vi "SimpleScanning_August12_2016.vi"() -> ()   [LabVIEW 2010]
uses:
  <vilib>/DAQmx/configure/timing.llb/DAQmx Timing (Sample Clock).vi
  <vilib>/Analysis/NI_AALBase.lvlib
  <vilib>/DAQmx/create/channels.llb/DAQmx Create Channel (AO-Voltage-Basic).vi
  <vilib>/DAQmx/configure/trigger.llb/DAQmx Start Trigger (Digital Edge).vi
  <vilib>/DAQmx/create/channels.llb/DAQmx Create Channel (AI-Voltage-Basic).vi
  <vilib>/DAQmx/read.llb/DAQmx Read (Analog 1D DBL 1Chan NSamp).vi
  <vilib>/DAQmx/write.llb/DAQmx Write (Analog 2D DBL NChan NSamp).vi
panel:
  in  "offset (V)":dbl=1000.0
  in  "display scaled image?":bool
  in  "Pixels (X,Y)":i32[](array[numeric])=[200, 200]
  in  "Scan amplitude (X,Y) (V)":dbl[](array[numeric])=[2.0, 2.0]
  out "min,max raw pixel voltage":dbl[](array[numeric])
  in  "scale factor":i32=1000
  in  "rescale pixel values":bool=TRUE
  out "Histogram Graph":T1(graph)
  out "Image Gr":dbl[][](graph)
  in  "Invert":bool=TRUE
  out "file path":path
  out "file #":i32
  in  "file tag":string="t"
  out "stop 2":bool
  in  "SAVE":bool
  in  "AI input\nconfiguration":i32(ring)=-1 items=["default"=-1, "RSE"=10083, "NRSE"=10078, "Differential"=10106, "Pseudodifferential"=12529]
  in  "refnum tif":refnum<file>
  in  "AI range (+/-) (V)":dbl=2.0 format="%#_13g"
  in  "AI rate (Hz): Max":dbl=4000000.0 format="%#_13g"
  in  "AO rate (Hz): Max":dbl=4000000.0 format="%#_13g"
  out "Array":dbl[][](array[numeric])
  out "Saved":i32
  in  "save local":bool
  in  "#frames":i32=10
  in  "Data Folder":path=path "C:/Users/TENSS/Desktop"
  out "Ypixels":i32=200
  in  "bidirectional":bool
  in  "samples to bin":i32=5
  out "current AI Rate (Hz)":dbl=2500000.0 format="%0.2f"
  in  "y flyback":bool=TRUE
  in  "stop":bool
  out "xy scan waveform":dbl[][](array[numeric])
  out "dwell time [us]":dbl=2.0
  in  "pixel shift":i32
  out "chunk to read":i32=1400
  out "input buffer size":i32=5000000
  in  "reset":bool
  out "#samples/frame":i32=56280
  out "Frame rate (hz)":dbl=8.884150675195452
  out "nlines":i32=200
  in  "flyback pixels (X)":i32=80
  out "Xpixels":i32=200
  in  "current AO Rate (Hz)":dbl=50000.0 format="%0.2f"
  # "Scan and Image assembly"
  # "DAQ related settings"
  # "Adjust scale factor, invert  to ensure the histogram\nspans large range 0-10000 or more\n--- efficiently use of the 16 bit dynamic range"
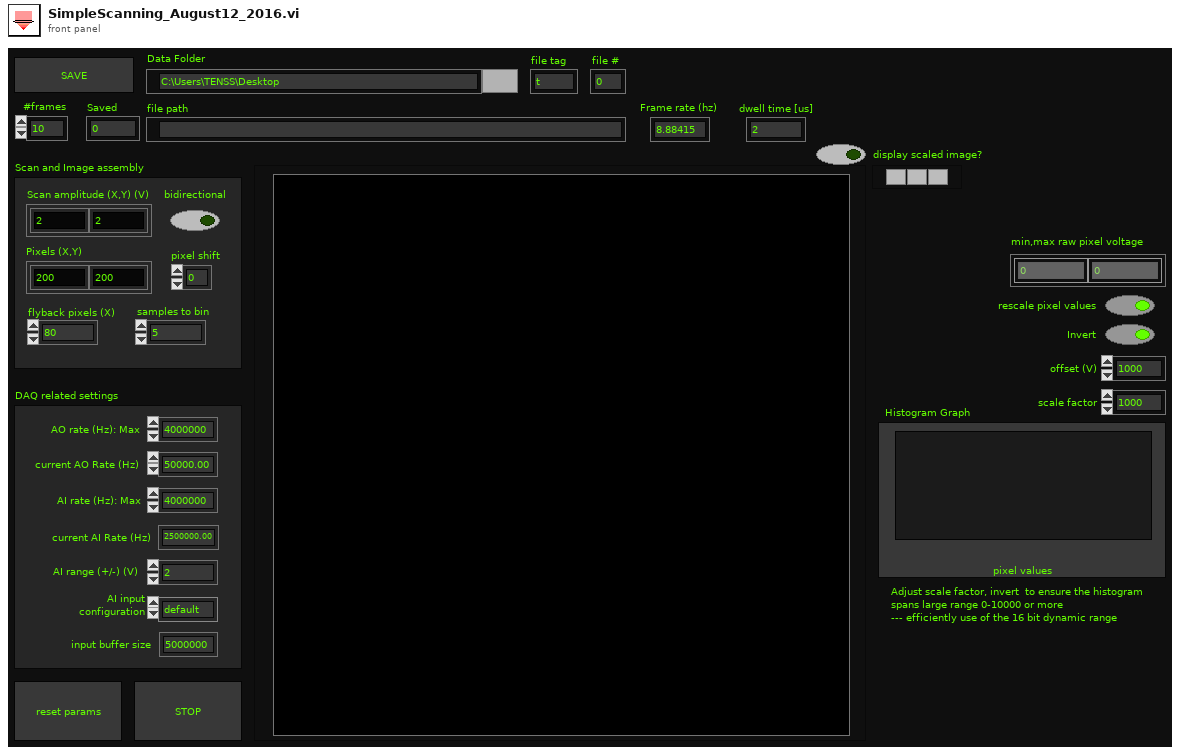
[diagram p1: front panel]
types:
  T1 = cluster{"X Values":dbl[], "Histogram: h(x)":i32[]}
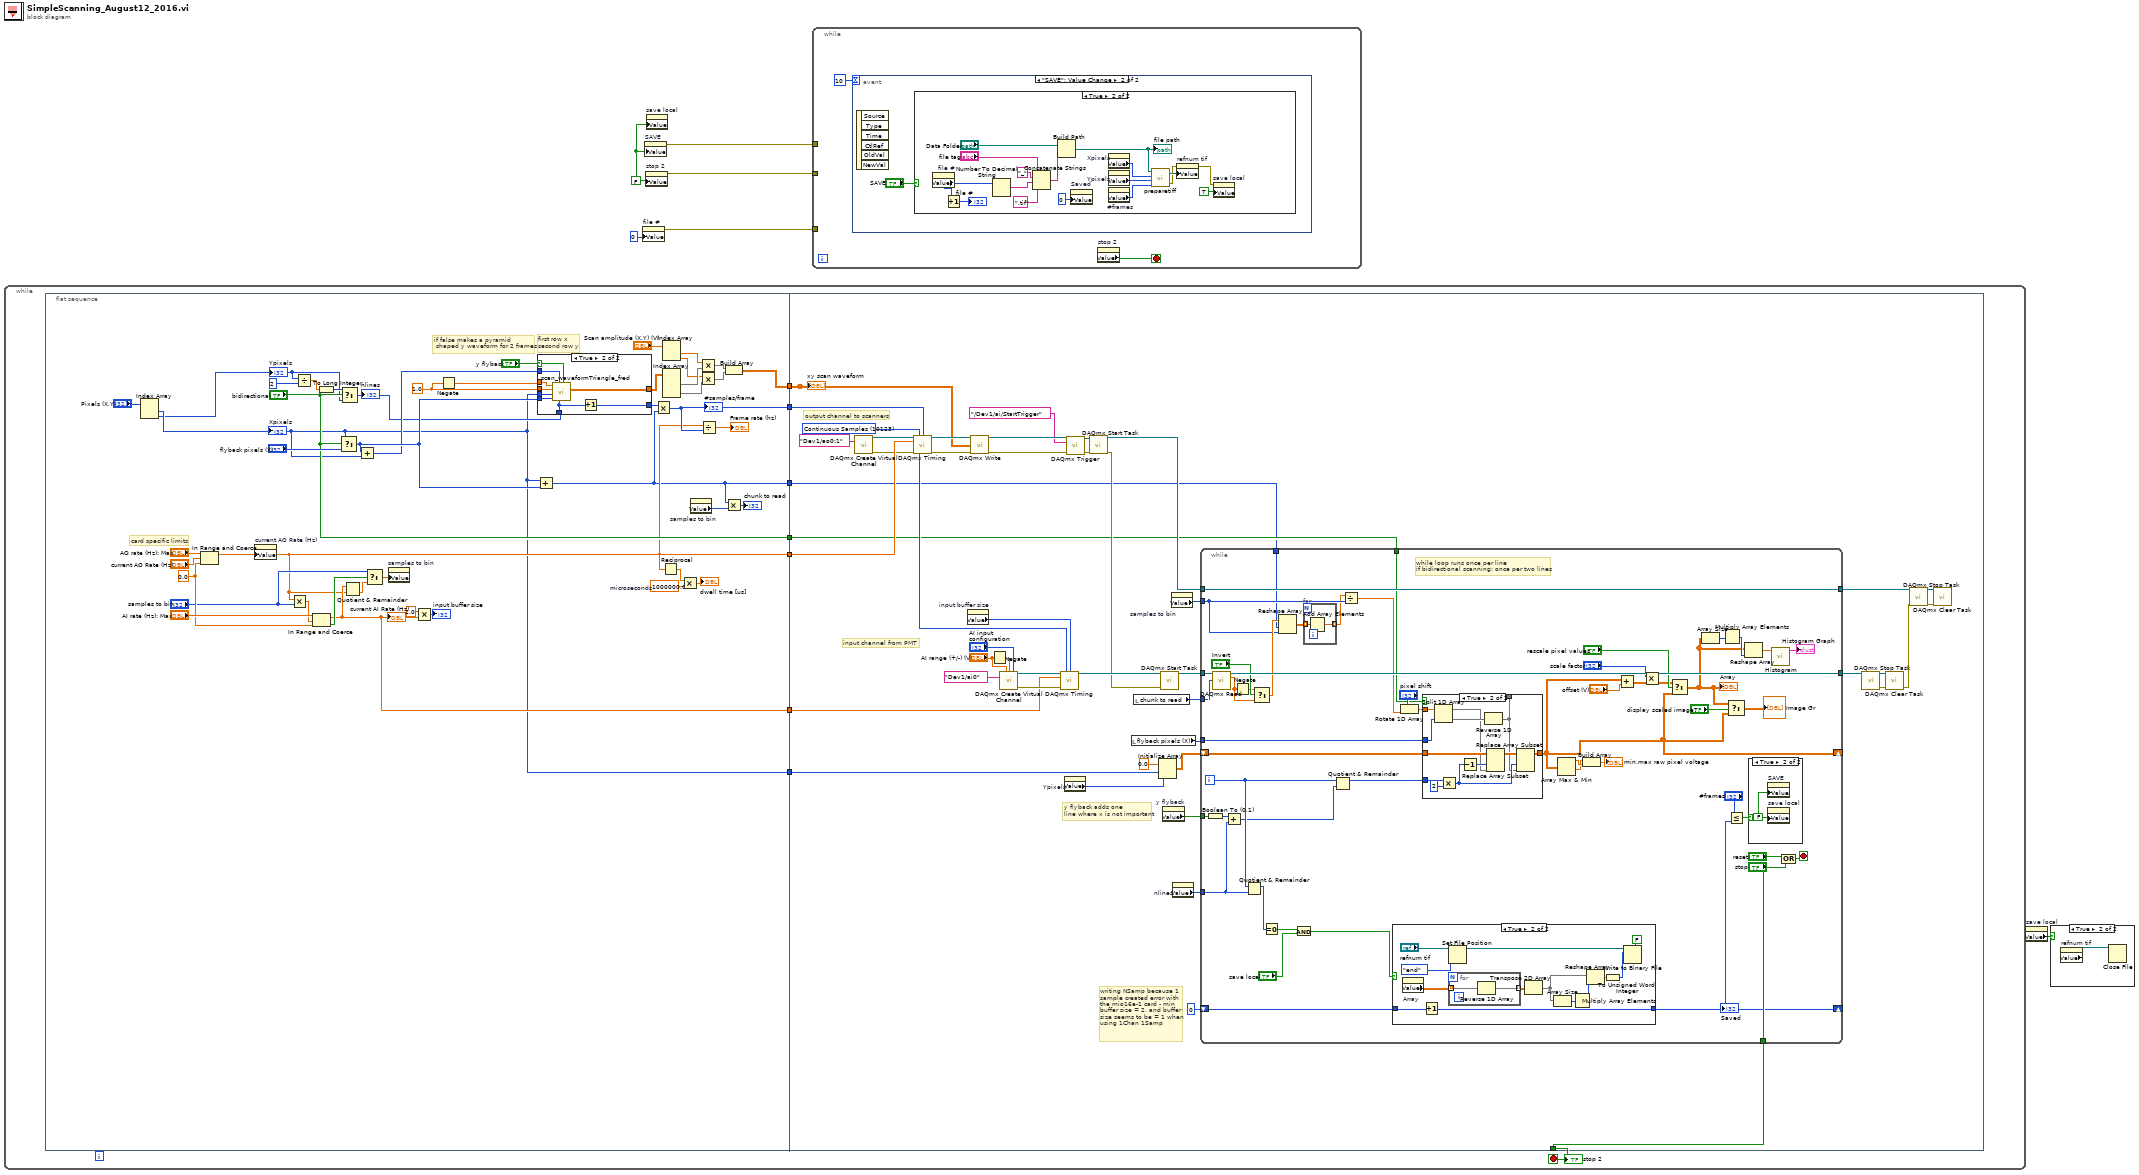
[diagram p0: block diagram]
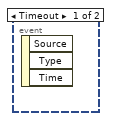
[diagram p2: hidden frame]
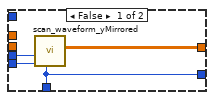
[diagram p5: hidden frame]
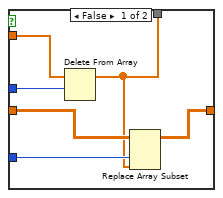
[diagram p8: hidden frame]
diagram:
  w4 = FALSE ("stop 2")
  n1 = while {
    stop <- w14 stop-if-true
    n2 = flat-sequence {
      tunnel: [w25] -> w13
      tunnel: [w43] -> w12
      tunnel: [w15] -> w11
      tunnel: [w29] -> w10
      tunnel: [w31] -> w9
      tunnel: ["bidirectional"] -> w8
      tunnel: [w28] -> w7
      tunnel: [w105] -> w14
      tunnel: w13 -> [w89]
      tunnel: w12 -> [w88]
      tunnel: w11 -> [w73]
      tunnel: w10 -> [w87]
      tunnel: w9 -> [w85]
      tunnel: w8 -> [w84]
      tunnel: w7 -> [w74]
      frame #0 {
        w27 = 1.0 ("scan voltage")
        w38 = 0.0 ("lower limit")
        w45 = 1000000.0  # microseconds
        # "card specific limits"
        # "first row x\nsecond row y"
        # "if false makes a pyramid\n shaped y waveform for 2 frames"
        n3 = Index Array(array="Pixels (X,Y)") -> (element #1=w25:i32, element #2=w24:i32)  [unwired: 2 in]
        "Xpixels" <- w25
        "Ypixels" <- w24
        n4 = In Range and Coerce(upper limit="AO rate (Hz): Max", x="current AO Rate (Hz)", lower limit=w38) -> (coerced(x)=w29:dbl)  [unwired: 1 out]
        n5 = property on="current AO Rate (Hz)" class="DigNum (strict)"("Value"=w29) -> ()  [unwired: 2 in, 2 out]
        n6 = Multiply(x=w29, y="samples to bin") -> (x*y=w37:dbl)
        n7 = Divide(x=w24, y=2) -> (x/y=w52:dbl)
        n8 = In Range and Coerce(upper limit="AI rate (Hz): Max", x=w37, lower limit=w38) -> (coerced(x)=w31:dbl, In Range?=w36:bool)
        "current AI Rate (Hz)" <- w31
        n9 = To Long Integer(number=w52) -> (32bit integer=w47:i32)
        n10 = Select(t=w25, s="bidirectional", f="flyback pixels (X)") -> (s? t:f=w50:i32)
        n11 = Select(t=w47, s="bidirectional", f=w24) -> (s? t:f=w48:i32)
        "nlines" <- w48
        n12 = Quotient & Remainder(x=w31, y=w29) -> (floor(x/y)=w34:dbl)  [unwired: 1 out]
        n13 = Add(x=w50, y=w25) -> (x+y=w49:i32)
        n14 = Select(t="samples to bin", s=w36, f=w34) -> (s? t:f=w33:dbl)
        n15 = property on="samples to bin" class="DigNum (strict)"("Value"=w33) -> ()  [unwired: 2 in, 2 out]
        n16 = Multiply(x=2.0 ("y"), y=w31) -> (x*y=→"input buffer size":dbl)
        n17 = Negate(x=w27) -> (-x=w55:dbl)
        n18 = case shown="True" "y flyback" {
          selector: "y flyback" -> [_ w66]
          tunnel: w48 -> [w60 w65]
          tunnel: [w63 w70] -> w23
          tunnel: w50 -> [w62 w72]
          tunnel: w25 -> [w61 w71]
          tunnel: w55 -> [_ w69]
          tunnel: w27 -> [_ w68]
          tunnel: w49 -> [_ w67]
          tunnel: [w60 w64] -> w46
          frame False {
            n19 = call "scan_waveform_yMirrored.vi"("nlines"=w60, "flyback"=w62, "xpixels"=w61) -> ("xy scan waveform"=w63:dbl[][])  [unwired: 4 in, 4 out]
          }
          frame True {
            n20 = call "scan_waveformTriangle_fred.vi"(5:"y flyback"=w66, "nlines"=w65, 7:"y flyback"=w67, "flyback"=w72, "xpixels"=w71, "maxV"=w68, "minV"=w69) -> ("xy scan waveform"=w70:dbl[][])  [unwired: 4 out]
            n21 = Increment(x=w65) -> (x+1=w64:i32)
          }
        }
        n22 = Add(x=w25, y=w50) -> (x+y=w28:i32)
        n23 = Multiply(x=w46, y=w28) -> (x*y=w43:i32)
        "#samples/frame" <- w43
        n24 = Reciprocal(x=w29) -> (1/x=w32:dbl)
        n25 = Index Array(array="Scan amplitude (X,Y) (V)") -> (element #1=w21:dbl, element #2=w18:dbl)  [unwired: 2 in]
        n26 = Index Array(array=w23) -> (element #1=w19:dbl[], element #2=w20:dbl[])  [unwired: 4 in]
        n27 = Multiply(x=w32, y=w45) -> (x*y=→"dwell time [us]":dbl)
        n28 = property on="samples to bin" class="DigNum (strict)"() -> ("Value"=w44:i32)  [unwired: 2 in, 2 out]
        n29 = Multiply(x=w21, y=w19) -> (x*y=w17:dbl[])
        n30 = Multiply(x=w18, y=w20) -> (x*y=w16:dbl[])
        n31 = Divide(x=w29, y=w43) -> (x/y=→"Frame rate (hz)":dbl)
        n32 = Build Array(w17, w16) -> (w15:dbl[][])
        n33 = Multiply(x=w28, y=w44) -> (x*y=→"chunk to read":i32)
      }
      frame #1 {
        w86 = 10123 items=["Finite Samples"=10178, "Continuous Samples"=10123, "Hardware Timed Single Point"=12522] ("sample mode")
        # "writing NSamp because 1 sample created error with\nthe mio16e-1 card - min\nbuffer size = 2, and buffer size seems to be = 1 when using 1Chan 1Samp"
        # "y flyback adds one\nline where x is not important"
        # "input channel from PMT"
        # "output channel to scanners"
        n34 = call-poly <vilib>:"DAQmx Create Virtual Channel.vi"("physical channels"=tag "Dev1/ao0:1") -> ("task out"=w79:refnum<k21>, "error out"=w78:errorcluster)  [unwired: 13 in]
        n35 = call-poly <vilib>:"DAQmx Timing.vi"("task/channels in"=w79, "sample mode"=w86, "samples per channel"=w88, "rate"=w87, "error in"=w78) -> ("task out"=w118:refnum<k21>, "error out"=w103:errorcluster)  [unwired: 2 in, 7 out]
        n36 = property on="input buffer size" class="DigNum (strict)"() -> ("Value"=w96:i32)  [unwired: 2 in, 2 out]
        n37 = call-poly <vilib>:"DAQmx Write.vi"("task/channels in"=w118, "data"=w73, "error in"=w103) -> ("task out"=w102:refnum<k21>, "error out"=w100:errorcluster)  [unwired: 1 in, 10 out]
        n38 = Negate(x="AI range (+/-) (V)") -> (-x=w90:dbl)
        n39 = call-poly <vilib>:"DAQmx Create Virtual Channel.vi"("maximum value"="AI range (+/-) (V)", "minimum value"=w90, "input terminal configuration"="AI input\nconfiguration", "physical channels"=tag "Dev1/ai0") -> ("task out"=w114:refnum<k21>, "error out"=w113:errorcluster)  [unwired: 5 in, 5 out]
        n40 = call-poly <vilib>:"DAQmx Timing.vi"("task/channels in"=w114, "sample mode"=w86, "samples per channel"=w96, "rate"=w85, "error in"=w113) -> ("task out"=w112:refnum<k21>)  [unwired: 2 in, 8 out]
        n41 = property on="Ypixels" class="DigNum (strict)"() -> ("Value"=w94:i32)  [unwired: 2 in, 2 out]
        n42 = call-poly <vilib>:"DAQmx Trigger.vi"("task/channels in"=w102, "source"=tag "/Dev1/ai/StartTrigger", "error in"=w100) -> ("task out"=w101:refnum<k21>, "error out"=w99:errorcluster)  [unwired: 1 in, 10 out]
        n43 = call <vilib>:"DAQmx Start Task.vi"("task/channels in"=w101, "error in"=w99) -> ("task out"=w117:refnum<k21>, "error out"=w98:errorcluster)  [unwired: 12 out]
        n44 = local read "flyback pixels (X)"() -> (w95:i32)
        n45 = local read "chunk to read"() -> (w106:i32)
        n46 = Initialize Array(0.0 ("element"), w89, w94) -> (w107:dbl[][])
        n47 = call <vilib>:"DAQmx Start Task.vi"("task/channels in"=w112, "error in"=w98) -> ("task out"=w111:refnum<k21>)  [unwired: 13 out]
        n48 = property on="y flyback" class="Bool (strict)"() -> ("Value"=w104:bool)  [unwired: 2 in, 2 out]
        n49 = property on="samples to bin" class="DigNum (strict)"() -> ("Value"=w97:i32)  [unwired: 2 in, 2 out]
        n50 = property on="nlines" class="DigNum (strict)"() -> ("Value"=w93:i32)  [unwired: 2 in, 2 out]
        n51 = while {
          tunnel: w117 -> [w169]
          tunnel: [w169] -> w116
          tunnel: w111 -> [w168]
          tunnel: [w167] -> w109
          tunnel: w106 -> [w166]
          tunnel: w95 -> [w165]
          shift-right: [w124] -> _
          shift-left: w107 -> [w157]
          tunnel: w93 -> [w148]
          tunnel: ["stop"] -> w105
          tunnel: w104 -> [w160]
          tunnel: w97 -> [w135]
          tunnel: w84 -> [w158]
          shift-right: [w155] -> _
          shift-left: 0 ("Border Size") -> [w156]
          tunnel: w74 -> [w134]
          i -> [w153]
          stop <- w163 stop-if-true
          # "while loop runs once per line\nif bidirectional scanning: once per two lines"
          n52 = Boolean To (0,1)(Boolean=w160) -> (0, 1=w150:i16)
          n53 = call-poly <vilib>:"DAQmx Read.vi"("task/channels in"=w168, "number of samples per channel"=w166) -> ("task out"=w167:refnum<k21>, "data"=w137:dbl[])  [unwired: 1 in, 11 out]
          n54 = Add(x=w150, y=w148) -> (x+y=w149:i32)
          n55 = Negate(x=w137) -> (-x=w144:dbl[])
          n56 = Quotient & Remainder(x=w153, y=w148) -> (x-y*floor(x/y)=w152:i32)  [unwired: 1 out]
          n57 = Select(t=w144, s="Invert", f=w137) -> (s? t:f=w136:dbl[])
          n58 = Equal To 0?(x=w152) -> (x = 0?=w129:bool)
          n59 = Reshape Array(w136, w134, w135) -> (w133:dbl[][])
          n60 = And(x=w129, y="save local") -> (x .and. y?=w126:bool)
          n61 = for {
            tunnel: w133 -> [w187] mode=indexing
            tunnel: [w186] -> w132 mode=indexing
            n62 = Add Array Elements(numeric array=w187) -> (sum=w186:dbl)
          }
          n63 = Quotient & Remainder(x=w153, y=w149) -> (x-y*floor(x/y)=w154:i32)  [unwired: 1 out]
          n64 = Divide(x=w132, y=w135) -> (x/y=w145:dbl[])
          n65 = case shown="True" w126 {
            tunnel: w156 -> [w170 w180]
            tunnel: [w170 w179] -> w155
            frame False {
            }
            frame True {
              n66 = property on="Array" class="Arr (strict)"() -> ("Value"=w171:dbl[][])  [unwired: 2 in, 2 out]
              n67 = Increment(x=w180) -> (x+1=w179:i32)
              n68 = Set File Position(refnum="refnum tif", from (0:start)=enum16{"start", "end", "current"}."end") -> (refnum out=w183:refnum<file>)  [unwired: 1 in, 2 out]
              n69 = for {
                tunnel: w171 -> [w185] mode=indexing
                tunnel: [w184] -> w173 mode=indexing
                n70 = Reverse 1D Array(array=w185) -> (reversed array=w184:dbl[])
              }
              n71 = Transpose 2D Array(2D array=w173) -> (transposed array=w172:dbl[][])
              n72 = Array Size(array=w172) -> (size(s)=w178:i32[])
              n73 = Multiply Array Elements(1:w178) -> (0:w177:i32)
              n74 = Reshape Array(w172, w177) -> (w176:dbl[])
              n75 = To Unsigned Word Integer(number=w176) -> (unsigned 16bit integer=w175:u16[])
              n76 = Write to Binary File(file (use dialog)=w183, data=w175, 5:FALSE ("prepend array or string size? (T)")) -> ()  [unwired: 2 in, 4 out]
            }
          }
          "Saved" <- w155
          n77 = Rotate 1D Array(1:w145, 2:"pixel shift") -> (0:w164:dbl[])
          n78 = case shown="True" w158 {
            tunnel: w165 -> [w194 w204]
            tunnel: w164 -> [w193 w206]
            tunnel: w157 -> [w192 w201]
            tunnel: [w191 w197] -> w124
            tunnel: w154 -> [w190 w202]
            tunnel: [w189 w195] -> _
            frame False {
              n79 = Delete From Array(array=w193, length=w194) -> (array with subset deleted=w189:dbl[])  [unwired: 1 in, 1 out]
              n80 = Replace Array Subset(array=w192, new element=w189, index (col)=w190) -> (w191:dbl[][])  [unwired: 1 in]
            }
            frame True {
              n81 = Split 1D Array(array=w206, index=w204) -> (first subarray=w196:dbl[], second subarray=w205:dbl[])
              n82 = Multiply(x=w202, y=2) -> (x*y=w198:i32)
              n83 = Decrement(x=w198) -> (x-1=w200:i32)
              n84 = Reverse 1D Array(array=w205) -> (reversed array=w195:dbl[])
              n85 = Replace Array Subset(array=w201, new element=w196, index (col)=w200) -> (w199:dbl[][])  [unwired: 1 in]
              n86 = Replace Array Subset(array=w199, new element=w195, index (col)=w198) -> (w197:dbl[][])  [unwired: 1 in]
            }
          }
          n87 = Array Max & Min(array=w124) -> (max value=w120:dbl, min value=w119:dbl)  [unwired: 2 out]
          n88 = Build Array(w119, w120) -> (→"min,max raw pixel voltage":dbl[])
          n89 = Add(x=w124, y="offset (V)") -> (x+y=w138:dbl[][])
          n90 = Multiply(x="scale factor", y=w138) -> (x*y=w125:dbl[][])
          n91 = Select(t=w125, s="rescale pixel values", f=w124) -> (s? t:f=w123:dbl[][])
          "Array" <- w123
          n92 = Array Size(array=w123) -> (size(s)=w141:i32[])
          n93 = Multiply Array Elements(1:w141) -> (0:w140:i32)
          n94 = Select(t=w123, s="display scaled image?", f=w124) -> (s? t:f=→"Image Gr":dbl[][])
          n95 = Less Or Equal?(x="#frames", y=w155) -> (x <= y?=w147:bool)
          n96 = Reshape Array(w123, w140) -> (w139:dbl[])
          n97 = case shown="True" w147 {
            frame False {
            }
            frame True {
              w188 = FALSE
              n98 = property on="SAVE" class="Bool (strict)"("Value"=w188) -> ()  [unwired: 2 in, 2 out]
              n99 = property on="save local" class="Bool (strict)"("Value"=w188) -> ()  [unwired: 2 in, 2 out]
            }
          }
          n100 = call <vilib>:"Histogram.vi"("X"=w139) -> ("Histogram Graph"=→"Histogram Graph":T1)  [unwired: 7 in, 3 out]
          n101 = Compound Arithmetic op=OR("reset", "stop") -> (w163:bool)
        }
        n102 = call <vilib>:"DAQmx Stop Task.vi"("task/channels in"=w109) -> ("task out"=w110:refnum<k21>, "error out"=w83:errorcluster)  [unwired: 1 in, 12 out]
        n103 = call <vilib>:"DAQmx Clear Task.vi"("task in"=w110, "error in"=w83) -> ("error out"=w82:errorcluster)  [unwired: 13 out]
        n104 = call <vilib>:"DAQmx Stop Task.vi"("task/channels in"=w116, "error in"=w82) -> ("task out"=w115:refnum<k21>, "error out"=w81:errorcluster)  [unwired: 12 out]
        n105 = call <vilib>:"DAQmx Clear Task.vi"("task in"=w115, "error in"=w81) -> ()  [unwired: 14 out]
        "xy scan waveform" <- w73
      }
    }
    "stop 2" <- w14
  }
  n106 = property on="file #" class="DigNum (strict)"("Value"=0 ("file number")) -> (error out=w2:errorcluster)  [unwired: 2 in, 1 out]
  n107 = property on="SAVE" class="Bool (strict)"("Value"=w4) -> (error out=w3:errorcluster)  [unwired: 2 in, 1 out]
  n108 = property on="stop 2" class="Bool (strict)"("Value"=w4) -> (error out=w1:errorcluster)  [unwired: 2 in, 1 out]
  n109 = property on="save local" class="Bool (strict)"("Value"=w4) -> ()  [unwired: 2 in, 2 out]
  n110 = while {
    tunnel: w3 -> [_]
    tunnel: w2 -> [_]
    tunnel: w1 -> [_]
    stop <- w207 stop-if-true
    n111 = event shown="[1] \"SAVE\": Value Change" {
      selector: _ -> [_ _]
      dyn-events: _ -> [_ _]
      timeout: 10 -> [_ _]
      event Timeout {
        n112 = event-data() -> ()  [unwired: 1 in, 3 out]
      }
      event "SAVE": Value Change {
        n113 = event-data() -> ()  [unwired: 1 in, 6 out]
        n114 = case shown="True" "SAVE" {
          frame False {
          }
          frame True {
            n115 = property on="file #" class="DigNum (strict)"() -> ("Value"=w211:i32)  [unwired: 2 in, 2 out]
            n116 = Increment(x=w211) -> (x+1=→"file #":i32)
            n117 = Number To Decimal String(number=w211) -> (decimal integer string=w219:string)  [unwired: 1 in]
            n118 = Concatenate Strings("file tag", "_" ("string"), w219, ".tif" ("string")) -> (w215:string)
            n119 = Build Path(base path="Data Folder", name or relative path=w215) -> (appended path=w214:path)
            "file path" <- w214
            n120 = property on="Saved" class="DigNum (strict)"("Value"=0 ("Saved")) -> ()  [unwired: 2 in, 2 out]
            n121 = property on="Xpixels" class="DigNum (strict)"() -> ("Value"=w224:i32)  [unwired: 2 in, 2 out]
            n122 = property on="Ypixels" class="DigNum (strict)"() -> ("Value"=w225:i32)  [unwired: 2 in, 2 out]
            n123 = property on="#frames" class="DigNum (strict)"() -> ("Value"=w226:i32)  [unwired: 2 in, 2 out]
            n124 = call "preparetiff.vi"("z"=w226, "y"=w225, "x"=w224, "file path"=w214) -> ("error out"=w221:errorcluster, "refnum tif"=w223:refnum<file>)
            n125 = property on="refnum tif" class="Ref (strict)"(error in=w221, "Value"=w223) -> (error out=w220:errorcluster)  [unwired: 1 in, 1 out]
            n126 = property on="save local" class="Bool (strict)"(error in=w220, "Value"=TRUE ("save local")) -> ()  [unwired: 1 in, 2 out]
          }
        }
      }
    }
    n127 = property on="stop 2" class="Bool (strict)"() -> ("Value"=w207:bool)  [unwired: 2 in, 2 out]
  }
  n128 = property on="save local" class="Bool (strict)"() -> ("Value"=w6:bool)  [unwired: 2 in, 2 out]
  n129 = case shown="True" w6 {
    frame False {
    }
    frame True {
      n130 = property on="refnum tif" class="Ref (strict)"() -> ("Value"=w227:refnum<file>)  [unwired: 2 in, 2 out]
      n131 = Close File(refnum=w227) -> ()  [unwired: 1 in, 2 out]
    }
  }
